vi "Open.vi"(8 "error in (no error)":errorcluster, 11 "SV B-M (Target) in":refnum<class "SV B-M (Target).lvclass">) -> (0 "error out":errorcluster, 3 "SV B-M (Target) out":refnum<class "SV B-M (Target).lvclass">)   [LabVIEW 2015, in "SV B-M (Target).lvclass"]
uses:
  SV B-M (Target).lvclass
  SV B-M (Target).lvclass/SV B-M (Target).ctl
  Command & Ack - Send Ack.vi
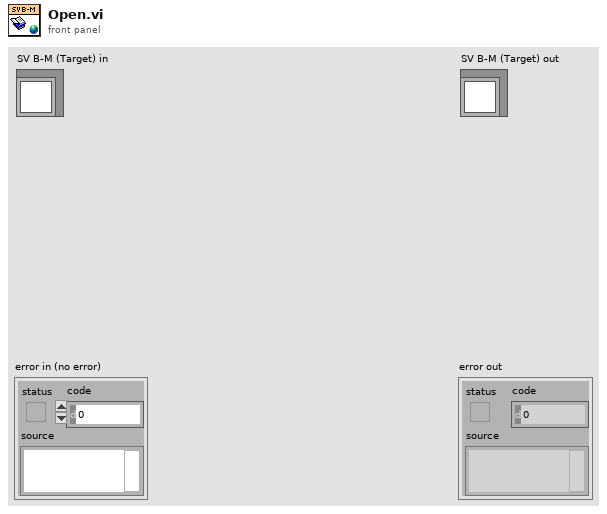
[diagram p1: front panel]
types:
  T1 = typedef "Variable Data Type.ctl" = enum16{"U8", "U16", "U32", "U64", "I8", "I16", "I32", "I64", "Single", "Double", "Boolean", "String"}
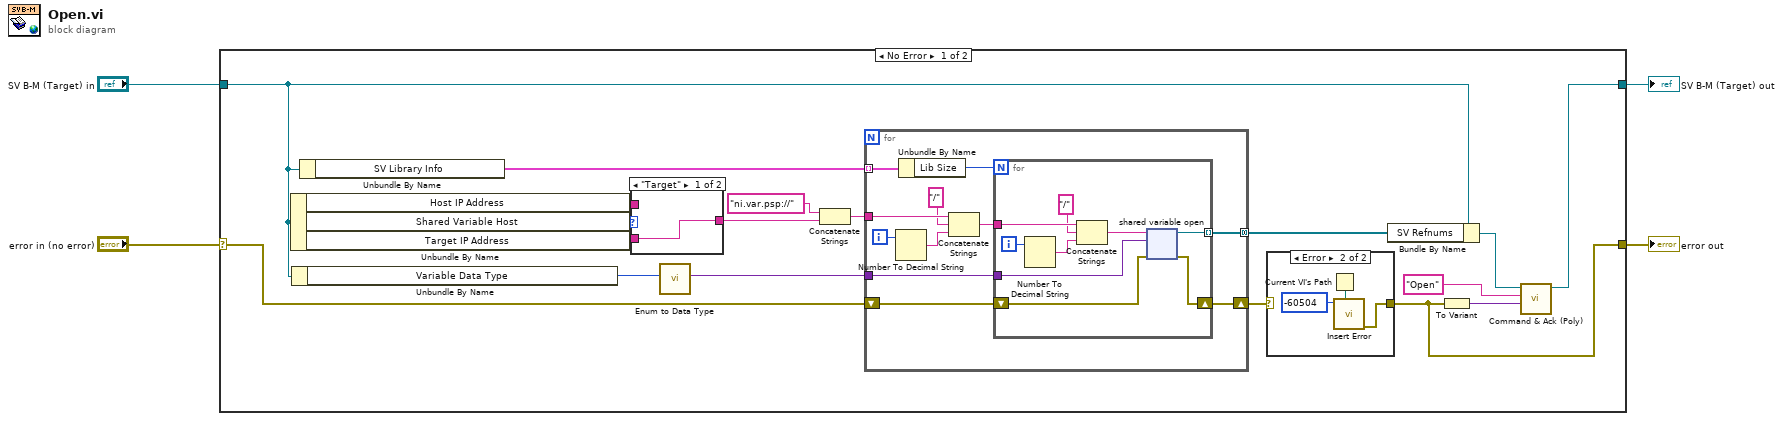
[diagram p0: block diagram]
diagram:
  n1 = case shown="No Error" "error in (no error)" {
    selector: "error in (no error)" -> [w13 w50]
    tunnel: [w5 w50] -> w3
    tunnel: [w8 w49] -> w1
    tunnel: "SV B-M (Target) in" -> [w12 w49]
    frame No Error {
      n2 = Unbundle By Name(w12) -> ("Host IP Address"=w17:string, "Shared Variable Host"=w16:enum16{"Target", "Host"}, "Target IP Address"=w15:string)
      n3 = Unbundle By Name(w12) -> ("Variable Data Type"=w14:T1)
      n4 = Unbundle By Name(w12) -> ("SV Library Info"=w18:cluster{"Lib Path":path, "Lib Size":u16}[])
      n5 = case shown="\"Target\"" w16 {
        tunnel: w17 -> [_ w28]
        tunnel: w15 -> [w27 _]
        tunnel: [w27 w28] -> w19
        frame "Target" {
        }
        frame "Host" {
        }
      }
      n6 = call "Enum to Data Type.vi"("Variable Data Type"=w14) -> ("Variant"=w22:variant)  [unwired: 10 in]
      n7 = Concatenate Strings("ni.var.psp://", w19) -> (w21:string)
      n8 = for {
        tunnel: w18 -> [w39] mode=indexing
        tunnel: w21 -> [w37]
        shift-right: [w29] -> w6
        shift-left: w13 -> [w32]
        tunnel: w22 -> [w31]
        tunnel: [w30] -> w7 mode=concatenating
        i -> [w36]
        n9 = Number To Decimal String(number=w36) -> (decimal integer string=w35:string)  [unwired: 1 in]
        n10 = Unbundle By Name(w39) -> ("Lib Size"=w38:u16)
        n11 = Concatenate Strings(w37, "/", w35) -> (w33:string)
        n12 = for {
          N: w38 -> [_]
          tunnel: w33 -> [w47]
          shift-right: [w41] -> w29
          shift-left: w32 -> [w43]
          tunnel: w31 -> [w42]
          tunnel: [w40] -> w30 mode=indexing
          i -> [w48]
          n13 = Number To Decimal String(number=w48) -> (decimal integer string=w46:string)  [unwired: 1 in]
          n14 = Concatenate Strings(w47, "/", w46) -> (w44:string)
          n15 = shared-variable-open(w44, w43, w42) -> (w40:refnum<k21>, w41:errorcluster)  [unwired: 2 in]
        }
      }
      n16 = case shown="Error" w6 {
        selector: w6 -> [w23 _]
        tunnel: [w23 w26] -> w5
        frame No Error {
        }
        frame Error {
          n17 = Current VI's Path() -> (path=w24:path)
          n18 = call "Insert Error.vi"("VI Path"=w24, "Error Code"=-60504) -> ("error out"=w26:errorcluster)  [unwired: 9 in]
        }
      }
      n19 = Bundle By Name(cluster=w12, "SV Refnums"=w7) -> (w11:refnum<class "SV B-M (Target).lvclass">)
      n20 = To Variant(anything=w5) -> (Variant=w10:variant)
      n21 = call-poly "Command & Ack (Poly).vi"("Message Data"=w10, "Message"="Open", "SV B-M (Target) In"=w11) -> ("SV B-M (Target) Out"=w8:refnum<class "SV B-M (Target).lvclass">)  [unwired: 6 in, 2 out]
    }
    frame Error {
    }
  }
  "error out" <- w3
  "SV B-M (Target) out" <- w1
